vi "Register for Folder Path.vi"(8 "error in (no error)":errorcluster, 11 "Test Executive Explorer in":refnum<class "Test Executive Explorer.lvclass">) -> (0 "error out":errorcluster, 3 "Test Executive Explorer out":refnum<class "Test Executive Explorer.lvclass">)   [LabVIEW 2017, in "Test Executive Explorer.lvclass"]
uses:
  Test Executive Explorer.lvclass
  <vilib>/gpm_packages/@cs/file-explorer-extension/Source/File Explorer/File Explorer/File Explorer.lvclass
  C:/Users/jonmc/Documents/Git/Test Executive Builder/gpm_packages/@cs/file-explorer-extension/Source/File Explorer/File Explorer/File Explorer.lvclass
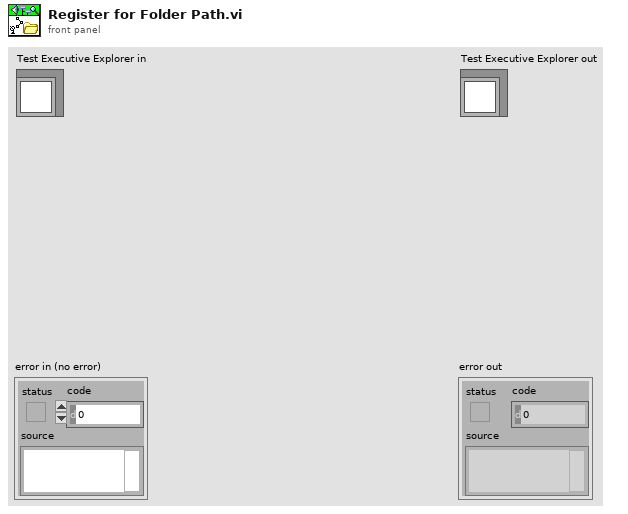
[diagram p1: front panel]
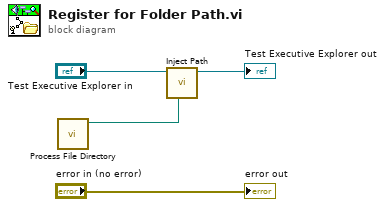
[diagram p0: block diagram]
diagram:
  n1 = call "Process File Directory.vi"() -> ("Process File Directory"=w1:path)  [unwired: 11 in]
  n2 = call <vilib>:"Inject Path.vi"("Path"=w1, "File Explorer in"="Test Executive Explorer in") -> ("File Explorer out"=→"Test Executive Explorer out":refnum<class "Test Executive Explorer.lvclass">)  [unwired: 9 in]
  "error out" <- "error in (no error)"
